vi "Generate Overlap SQL Query.vi"(8 "error in (no error)":errorcluster, 10 "Importing Transaction Count":i32, 11 "First Importing Transaction":refnum<class "Banking Record.lvclass">) -> (0 "error out":errorcluster, 2 "SELECT SQL Query":string, 3 "First Importing Transaction":refnum<class "Banking Record.lvclass">)   [LabVIEW 2018, in "Banking Record.lvclass"]
uses:
  Banking Record.lvclass
  Transaction/Transaction.lvclass
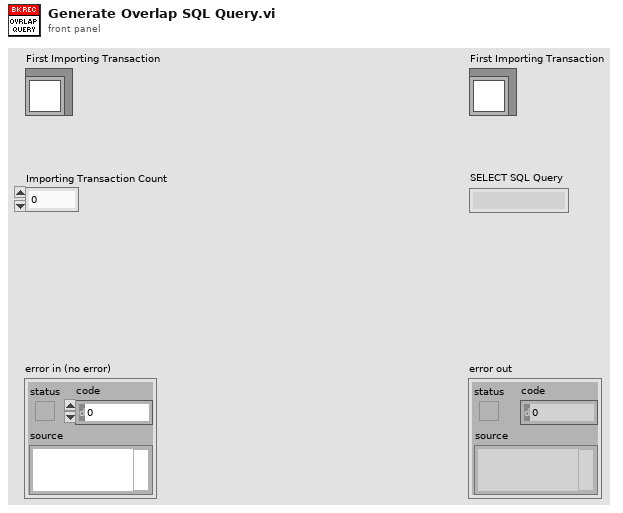
[diagram p1: front panel]
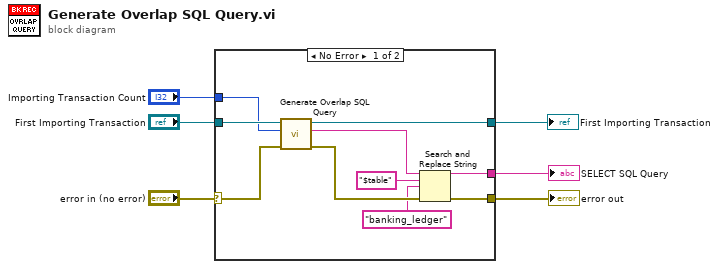
[diagram p0: block diagram]
diagram:
  n1 = case shown="No Error" "error in (no error)" {
    selector: "error in (no error)" -> [w7 w17]
    tunnel: "First Importing Transaction" -> [w16 w18]
    tunnel: "Importing Transaction Count" -> [w15 _]
    tunnel: [w14 w18] -> w4
    tunnel: [w9 w17] -> w3
    tunnel: [w8 _] -> w2
    frame No Error {
      n2 = call-parent "Generate Overlap SQL Query.vi"("error in (no error)"=w7, "num of csv transactions"=w15, "First Importing Transaction"=w16) -> ("error out"=w12:errorcluster, "SELECT SQL Query"=w13:string, "First Importing Transaction"=w14:refnum<class "Banking Record.lvclass">)  [unwired: 6 in]
      n3 = Search and Replace String(input string=w13, search string="$table", replace string="banking_ledger", error in=w12) -> (result string=w8:string, error out=w9:errorcluster)  [unwired: 4 in, 2 out]
    }
    frame Error {
    }
  }
  "error out" <- w3
  "First Importing Transaction" <- w4
  "SELECT SQL Query" <- w2
